vi "Update_Event_number.vi"(8 "error in (no error)":errorcluster, 10 "number":string, 11 "NPad2 in":refnum<class "NPad2.lvclass">) -> (0 "error out":errorcluster, 3 "NPad2 out":refnum<class "NPad2.lvclass">)   [LabVIEW 2020, in "NPad2.lvlib" / "NPad2.lvclass"]
uses:
  NPad2.lvclass
  NPad2.lvclass/NPad2.ctl
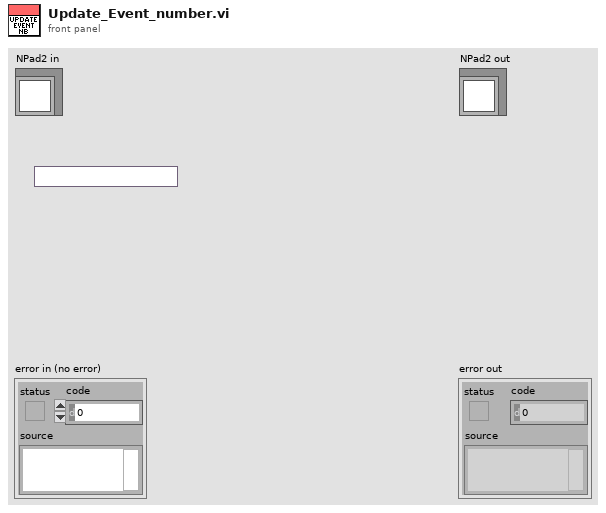
[diagram p1: front panel]
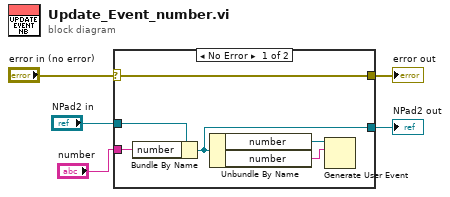
[diagram p0: block diagram]
diagram:
  n1 = case shown="No Error" "error in (no error)" {
    selector: "error in (no error)" -> [w11 w13]
    tunnel: [w11 w13] -> w4
    tunnel: [w8 w12] -> w2
    tunnel: "NPad2 in" -> [w10 w12]
    tunnel: "number" -> [w9 _]
    frame No Error {
      n2 = Bundle By Name(cluster=w10, "number"=w9) -> (w8:refnum<class "NPad2.lvclass">)
      n3 = Unbundle By Name(w8) -> ("number"=w7:refnum<user-event>, "number"=w6:string)
      n4 = Generate User Event(user event=w7, event data cluster=w6) -> ()  [unwired: 2 in, 2 out]
    }
    frame Error {
    }
  }
  "error out" <- w4
  "NPad2 out" <- w2
